vi "save as csv.vi"(8 "error in (no error)":errorcluster, 10 "csv path":path, 11 "Data Log in":refnum<class "Data Log.lvclass">) -> (0 "error out":errorcluster, 3 "Data Log out":refnum<class "Data Log.lvclass">)   [LabVIEW 2025, in "Data Log.lvclass"]
uses:
  Data Log.lvclass
  Data Log.lvclass/Data Log.ctl
  <vilib>/Utility/file.llb/Write Delimited Spreadsheet (DBL).vi
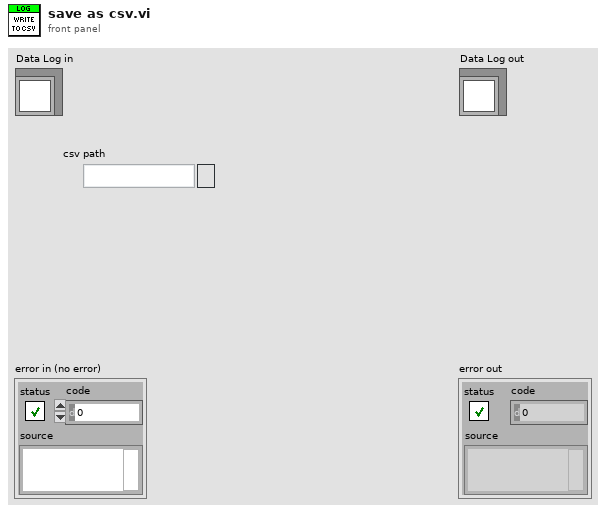
[diagram p1: front panel]
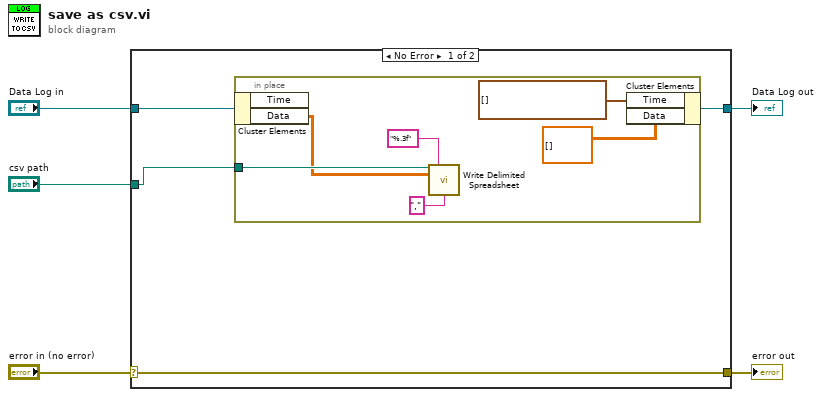
[diagram p0: block diagram]
diagram:
  n1 = case shown="No Error" "error in (no error)" {
    selector: "error in (no error)" -> [w9 w17]
    tunnel: [w9 w17] -> w4
    tunnel: [w7 w16] -> w2
    tunnel: "Data Log in" -> [w8 w16]
    tunnel: "csv path" -> [w6 _]
    frame No Error {
      n2 = in-place {
        in-place-border: w6 -> [w13]
        n3 = in-place-cluster #1(w8) -> ("Data"=w12:dbl[][])  [unwired: 1 out]
        n4 = call-poly <vilib>:"Write Delimited Spreadsheet.vi"("file path (dialog if empty)"=w13, "format (%.3f)"="%.3f", "2D data"=w12, "delimiter (\\t)"="," ("delimiter (\\t)")) -> ()  [unwired: 10 in, 2 out]
        n5 = in-place-cluster #1("Time"=timestamp[] [] ("Data.Time"), "Data"=dbl[][] [] ("Data.Data")) -> (w7:refnum<class "Data Log.lvclass">)
      }
    }
    frame Error {
    }
  }
  "error out" <- w4
  "Data Log out" <- w2
